vi "Main.vi"   [LabVIEW 2020, in "FormulaG.lvlib" / "FormulaG App.lvclass"]
uses:
  FormulaG App.lvclass
panel:
  # "FormulaG\nMain"
types:
  T1 = enum32{"Invalid", "Standard", "Closed", "Hidden", "Minimized", "Maximized"}
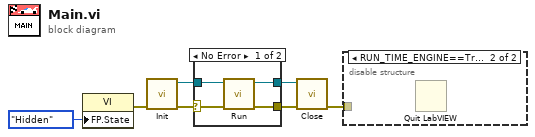
[diagram p0: block diagram]
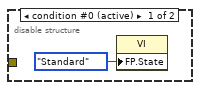
[diagram p2: hidden frame]
diagram:
  n1 = property class="VI"("FP.State"=T1."Hidden" ("Front Panel Window:State")) -> (error out=w6:errorcluster)  [unwired: 2 in, 1 out]
  n2 = call "Init.vi"("error in (no error)"=w6) -> ("error out"=w5:errorcluster, "FormulaLV App out"=w4:refnum<class "FormulaG App.lvclass">)  [unwired: 9 in]
  n3 = case shown="No Error" w5 {
    selector: w5 -> [w10 w13]
    tunnel: w4 -> [w11 w12]
    tunnel: [w9 w13] -> w3
    tunnel: [w8 w12] -> w2
    frame No Error {
      n4 = call "Run.vi"("error in (no error)"=w10, "FormulaLV App in"=w11) -> ("error out"=w9:errorcluster, "FormulaLV App out"=w8:refnum<class "FormulaG App.lvclass">)  [unwired: 8 in]
    }
    frame Error {
    }
  }
  n5 = call "Close.vi"("error in (no error)"=w3, "FormulaLV App in"=w2) -> ("error out"=w1:errorcluster)  [unwired: 9 in]
  n6 = disable-structure shown="RUN_TIME_ENGINE==True" {
    disable-tunnel: w1 -> [_ _]
    frame condition #0 (active) {
      n7 = property class="VI"("FP.State"=T1."Standard" ("Front Panel Window:State")) -> ()  [unwired: 2 in, 2 out]
    }
    frame condition #1 {
      n8 = Quit LabVIEW() -> ()  [unwired: 1 in]
    }
  }
